vi "axis_angle_to_quaternion.vi"(8 "Angle theta":dbl format="%.5f", 11 "Axis x":dbl[](array[numeric])) -> (3 "Quaternion":dbl[](array[numeric]))   [LabVIEW 2012]
uses:
  norm_vec.vi
panel:
  # "Given an axis vector and a rotation angle, return the unit quaternion for this 3D rotation."
  # "w"
  # "x1"
  # "x2"
  # "x3"
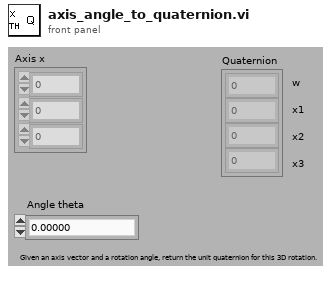
[diagram p1: front panel]
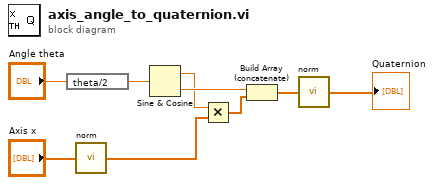
[diagram p0: block diagram]
diagram:
  n1 = expression code="theta/2"("Angle theta") -> (w7:dbl)
  n2 = call-poly "norm.vi"("vector"="Axis x") -> ("normalized vector"=w3:dbl[])  [unwired: 3 in, 1 out]
  n3 = Sine & Cosine(0:w7) -> (1:w4:dbl, 2:w6:dbl)
  n4 = Multiply(x=w4, y=w3) -> (x*y=w5:dbl[])
  n5 = Build Array (concatenate)(w6, w5) -> (w2:dbl[])
  n6 = call-poly "norm.vi"("vector"=w2) -> ("normalized vector"=→"Quaternion":dbl[])  [unwired: 3 in, 1 out]
